vi "Set Image Version.vi"(8 "error in (no error)":errorcluster, 10 "Image Version":string, 11 "Device in":refnum<class "Device.lvclass">=refnum) -> (0 "error out":errorcluster, 3 "Device out":refnum<class "Device.lvclass">)   [LabVIEW 2015]
uses:
  Device.lvclass
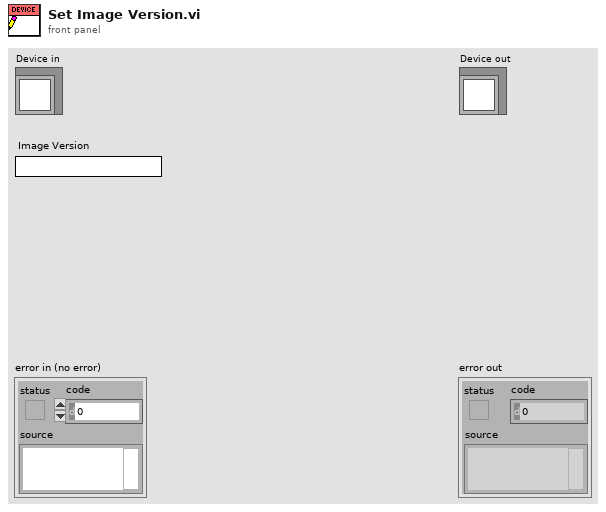
[diagram p1: front panel]
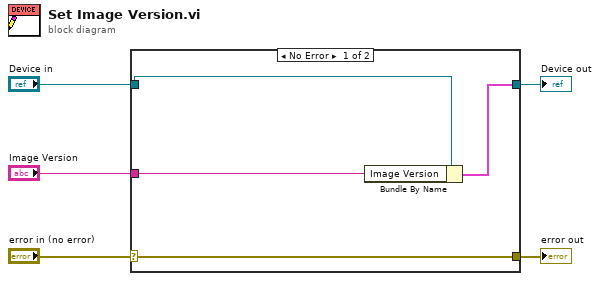
[diagram p0: block diagram]
diagram:
  n1 = case shown="No Error" "error in (no error)" {
    selector: "error in (no error)" -> [w9 w10]
    tunnel: [w9 w10] -> w4
    tunnel: [w7 w11] -> w2
    tunnel: "Device in" -> [w8 w11]
    tunnel: "Image Version" -> [w6 _]
    frame No Error {
      n2 = Bundle By Name(cluster=w8, "Image Version"=w6) -> (w7:cluster{})
    }
    frame Error {
    }
  }
  "error out" <- w4
  "Device out" <- w2
